vi "Form time_delays.vi"(8 "error in (no error)":errorcluster, 9 "remake":bool, 10 "Control-Client":refnum<class "Control-Client.lvclass">, 11 "Experiment in":refnum<class "Experiment.lvclass">) -> (0 "error out":errorcluster, 2 "Control-Client out":refnum<class "Control-Client.lvclass">, 3 "Experiment out":refnum<class "Experiment.lvclass">)   [LabVIEW 2018, in "Experiment.lvclass"]
uses:
  Experiment.lvclass
  Control/Control-Client/Control-Client.lvclass
  Experiment.lvclass/Experiment.ctl
  Control/Control-Client/Control-Client.lvclass/Control-Client.ctl
panel:
  out "minI":dbl
  out "Real Optical 0, ps":dbl
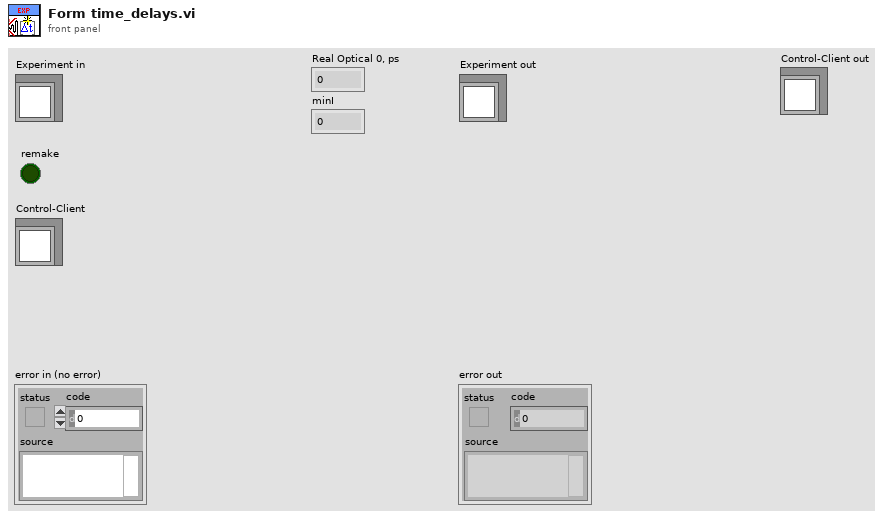
[diagram p1: front panel]
types:
  T1 = cluster{"min I, mm":dbl, "max I, mm":dbl, "Real Optical 0, ps":dbl, "min II, mm":dbl, "max II, mm ":dbl}
  T2 = typedef "Control-Client.lvclass/Delays-refs_CLIENT.ctl" = cluster{"# points":refnum<vi>, "Step, ps":refnum<vi>, "OZ, ps":refnum<vi>, "# current":refnum<vi>, "RDT, ps":refnum<vi>, "Total length, ps":refnum<vi>, "Kinetics length, ps":refnum<vi>, "Real zero, ps":refnum<vi>, "# par point":refnum<vi>}
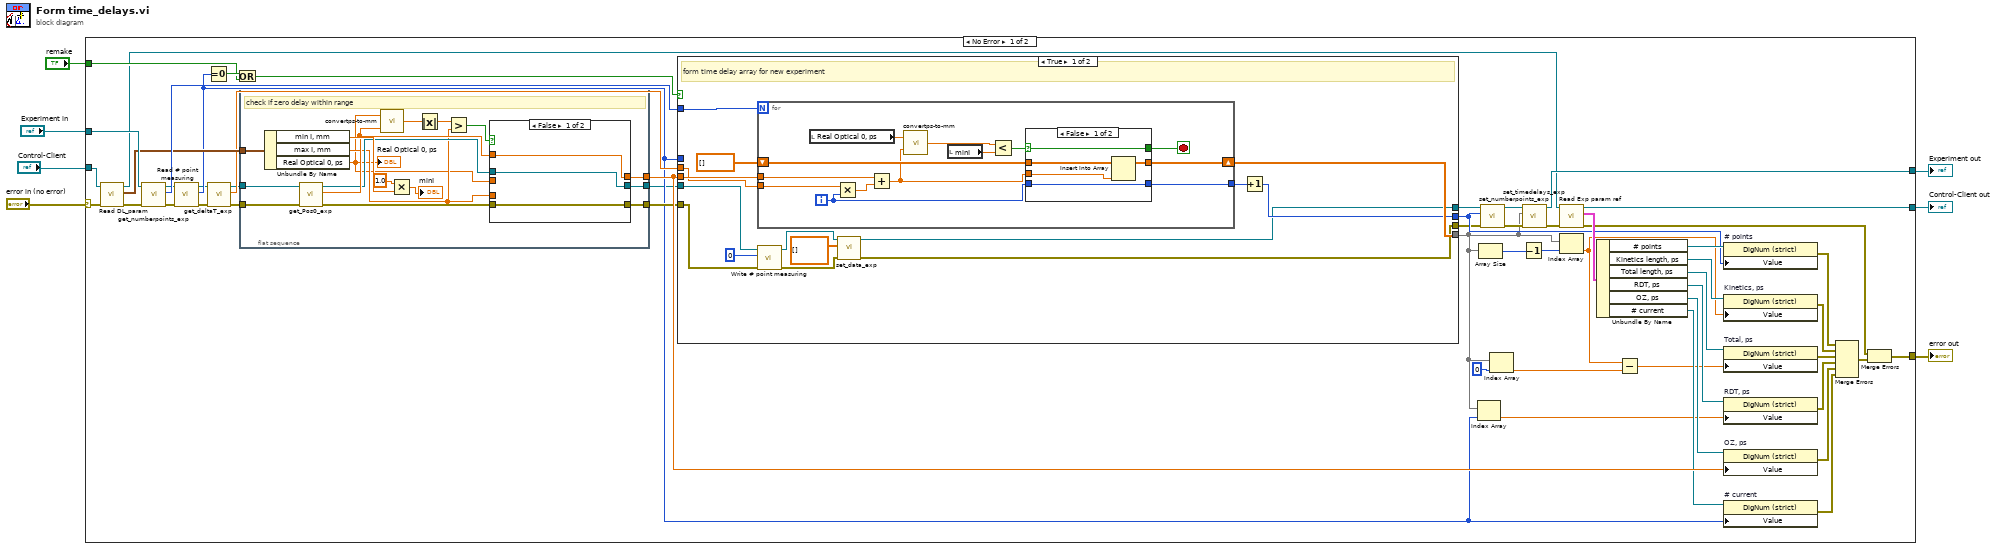
[diagram p0: block diagram]
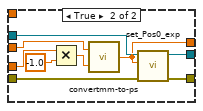
[diagram p2: hidden frame]
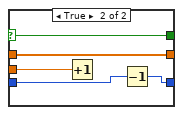
[diagram p3: hidden frame]
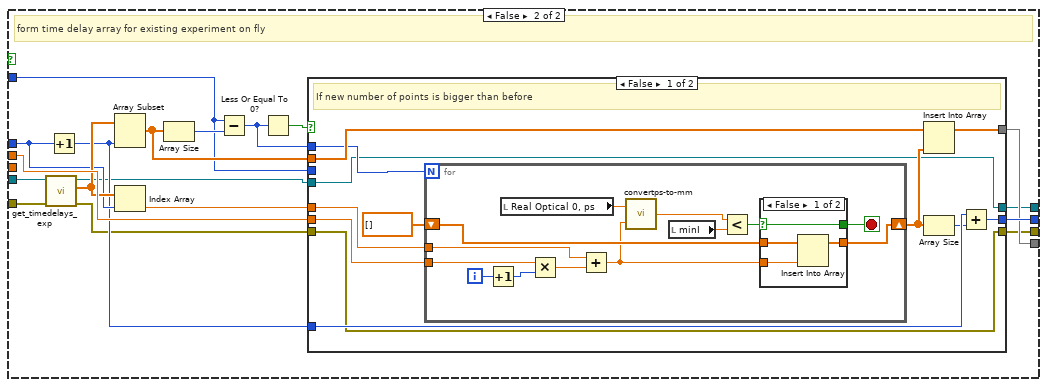
[diagram p4: hidden frame]
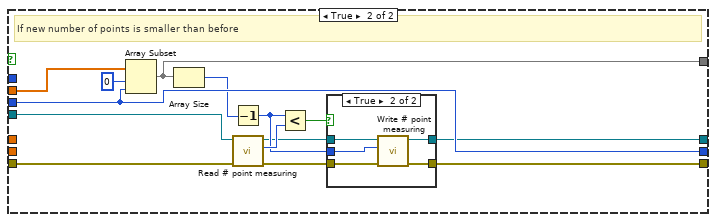
[diagram p6: hidden frame]
diagram:
  n1 = case shown="No Error" "error in (no error)" {
    selector: "error in (no error)" -> [w11 w200]
    tunnel: [w55 w200] -> w6
    tunnel: [w60 w199] -> w4
    tunnel: "Experiment in" -> [w56 w199]
    tunnel: "Control-Client" -> [w52 w198]
    tunnel: "remake" -> [w27 _]
    tunnel: [w18 w198] -> w1
    frame No Error {
      n2 = call "Read DL_param.vi"("error in (no error)"=w11, "Control-Client in"=w52) -> ("error out"=w10:errorcluster, "DL_param"=w54:T1, "Control-Client out"=w19:refnum<class "Control-Client.lvclass">)  [unwired: 7 in]
      n3 = call "get_numberpoints_exp.vi"("error in (no error)"=w10, "Experiment.lvclass in"=w56) -> ("error out"=w14:errorcluster, "numberpoints"=w59:i32, "Experiment.lvclass out"=w17:refnum<class "Experiment.lvclass">)  [unwired: 7 in]
      n4 = call "Read # point measuring.vi"("error in (no error)"=w14, "Experiment in"=w17) -> ("error out"=w13:errorcluster, "# point measuring"=w25:i32, "Experiment out"=w16:refnum<class "Experiment.lvclass">)  [unwired: 7 in]
      n5 = Equal To 0?(x=w25) -> (x = 0?=w29:bool)
      n6 = call "get_deltaT_exp.vi"("error in (no error)"=w13, "Experiment.lvclass in"=w16) -> ("error out"=w12:errorcluster, "deltaTlast"=w33:dbl, "Experiment.lvclass out"=w15:refnum<class "Experiment.lvclass">)  [unwired: 7 in]
      n7 = Or(x=w29, y=w27) -> (x .or. y?=w28:bool)
      n8 = flat-sequence {
        tunnel: w54 -> [w77]
        tunnel: [w70] -> w34
        tunnel: w15 -> [w67]
        tunnel: [w66] -> w23
        tunnel: [w63] -> w31
        tunnel: w12 -> [w61]
        frame #0 {
          # "check if zero delay within range"
          n9 = Unbundle By Name(w77) -> ("min I, mm"=w76:dbl, "max I, mm"=w65:dbl, "Real Optical 0, ps"=w64:dbl)
          "Real Optical 0, ps" <- w64
          n10 = call "get_Pos0_exp.vi"("error in (no error)"=w61, "Experiment.lvclass in"=w67) -> ("error out"=w68:errorcluster, "Delay0,ps"=w71:dbl, "Experiment.lvclass out"=w69:refnum<class "Experiment.lvclass">)  [unwired: 6 in]
          n11 = call "convertps-to-mm.vi"("ps"=w71, "Real zero"=w64) -> ("mm"=w74:dbl)
          n12 = Multiply(x=1.0, y=w76) -> (x*y=→"minI":dbl)
          n13 = Absolute Value(x=w74) -> (abs(x)=w73:dbl)
          n14 = Greater?(x=w73, y=w65) -> (0:w72:bool)
          n15 = case shown="False" w72 {
            tunnel: [w80 w83] -> w70
            tunnel: w71 -> [w80 _]
            tunnel: w69 -> [w79 w89]
            tunnel: w68 -> [w78 w88]
            tunnel: [w78 w87] -> w63
            tunnel: [w79 w86] -> w66
            tunnel: w65 -> [_ w84]
            tunnel: w64 -> [_ w85]
            frame False {
            }
            frame True {
              n16 = Multiply(x=w84, y=-1.0) -> (x*y=w82:dbl)
              n17 = call "convertmm-to-ps.vi"("mm"=w82, "Real zero"=w85) -> ("ps"=w83:dbl)
              n18 = call "set_Pos0_exp.vi"("error in (no error)"=w88, "Pos0,ps"=w83, "Experiment.lvclass in"=w89) -> ("error out"=w87:errorcluster, "Experiment.lvclass out"=w86:refnum<class "Experiment.lvclass">)  [unwired: 6 in]
            }
          }
        }
      }
      n19 = case shown="True" w28 {
        tunnel: w59 -> [w104 w134]
        tunnel: w34 -> [w103 _]
        tunnel: w33 -> [w102 w145]
        tunnel: [w98 w141] -> w50
        tunnel: [w100 w140] -> w38
        tunnel: w25 -> [_ w139]
        tunnel: w23 -> [w97 w144]
        tunnel: [w90 w131] -> w32
        tunnel: w31 -> [w96 w130]
        tunnel: [w93 w129] -> w30
        frame True {
          # "form time delay array for new experiment"
          n20 = for {
            N: w104 -> [_]
            tunnel: w103 -> [w117]
            tunnel: w102 -> [w116]
            tunnel: [w105] -> w99
            shift-right: [w107] -> w100
            shift-left: dbl[] [] ("array w/ subset deleted") -> [w109]
            i -> [w106]
            stop <- w110 stop-if-true
            n21 = local read "Real Optical 0, ps"() -> (w114:dbl)
            n22 = Multiply(x=w116, y=w106) -> (x*y=w115:dbl)
            n23 = Add(x=w117, y=w115) -> (x+y=w108:dbl)
            n24 = call "convertps-to-mm.vi"("ps"=w108, "Real zero"=w114) -> ("mm"=w113:dbl)
            n25 = local read "minI"() -> (w112:dbl)
            n26 = Less?(x=w113, y=w112) -> (x < y?=w111:bool)
            n27 = case shown="False" w111 {
              selector: w111 -> [w122 w127]
              tunnel: [w122 w127] -> w110
              tunnel: w109 -> [w121 w126]
              tunnel: w108 -> [w120 w125]
              tunnel: [w119 w126] -> w107
              tunnel: w106 -> [w118 w124]
              tunnel: [w118 w123] -> w105
              frame False {
                n28 = Insert Into Array(array=w121, new element=w120) -> (w119:dbl[])  [unwired: 1 in]
              }
              frame True {
                n29 = Increment(x=w125) -> ()  [unwired: 1 out]
                n30 = Decrement(x=w124) -> (x-1=w123:i32)
              }
            }
          }
          n31 = call "Write # point measuring.vi"("error in (no error)"=w96, "# point measuring"=0, "Experiment in"=w97) -> ("error out"=w94:errorcluster, "Experiment out"=w91:refnum<class "Experiment.lvclass">)  [unwired: 7 in]
          n32 = call "set_data_exp.vi"("error in (no error)"=w94, "Data"=dbl[][] [], "Experiment.lvclass in"=w91) -> ("error out"=w93:errorcluster, "Experiment.lvclass out"=w90:refnum<class "Experiment.lvclass">)  [unwired: 7 in]
          n33 = Increment(x=w99) -> (x+1=w98:i32)
        }
        frame False {
          # "form time delay array for existing experiment on fly"
          n34 = call "get_timedelays_exp.vi"("error in (no error)"=w130, "Experiment.lvclass in"=w144) -> ("error out"=w132:errorcluster, "timedelays"=w143:dbl[], "Experiment.lvclass out"=w133:refnum<class "Experiment.lvclass">)  [unwired: 7 in]
          n35 = Increment(x=w139) -> (x+1=w138:i32)
          n36 = Array Subset(array=w143, length=w138) -> (w137:dbl[])  [unwired: 1 in]
          n37 = Index Array(array=w143, index=w139) -> (element=w142:dbl)
          n38 = Array Size(array=w137) -> (size(s)=w136:i32)
          n39 = Subtract(x=w134, y=w136) -> (x-y=w135:i32)
          n40 = Less Or Equal To 0?(x=w135) -> (x <= 0?=w128:bool)
          n41 = case shown="False" w128 {
            tunnel: w145 -> [w157 _]
            tunnel: w142 -> [w155 _]
            tunnel: [w154 w188] -> w141
            tunnel: [w153 w186] -> w140
            tunnel: w138 -> [w152 _]
            tunnel: w137 -> [w149 w190]
            tunnel: w135 -> [w148 _]
            tunnel: w134 -> [_ w188]
            tunnel: w133 -> [w146 w187]
            tunnel: w132 -> [w147 w181]
            tunnel: [w146 w179] -> w131
            tunnel: [w147 w177] -> w129
            frame False {
              # "If new number of points is bigger than before"
              n42 = for {
                N: w148 -> [_]
                tunnel: w155 -> [w170]
                tunnel: w157 -> [w169]
                shift-right: [w160] -> w151
                shift-left: dbl[] [] -> [w162]
                i -> [w167]
                stop <- w158 stop-if-true
                n43 = Increment(x=w167) -> (x+1=w159:i32)
                n44 = local read "Real Optical 0, ps"() -> (w166:dbl)
                n45 = Multiply(x=w169, y=w159) -> (x*y=w168:dbl)
                n46 = Add(x=w170, y=w168) -> (x+y=w161:dbl)
                n47 = call "convertps-to-mm.vi"("ps"=w161, "Real zero"=w166) -> ("mm"=w165:dbl)
                n48 = local read "minI"() -> (w164:dbl)
                n49 = Less?(x=w165, y=w164) -> (x < y?=w163:bool)
                n50 = case shown="False" w163 {
                  selector: w163 -> [w174 w176]
                  tunnel: [w174 w176] -> w158
                  tunnel: w162 -> [w173 w175]
                  tunnel: w161 -> [w172 _]
                  tunnel: [w171 w175] -> w160
                  frame False {
                    n51 = Insert Into Array(array=w173, new element=w172) -> (w171:dbl[])  [unwired: 1 in]
                  }
                  frame True {
                  }
                }
              }
              n52 = Insert Into Array(array=w149, new element=w151) -> (w153:dbl[])  [unwired: 1 in]
              n53 = Array Size(array=w151) -> (size(s)=w150:i32)
              n54 = Add(x=w152, y=w150) -> (x+y=w154:i32)
            }
            frame True {
              # "If new number of points is smaller than before"
              n55 = Array Subset(array=w190, index=0, length=w188) -> (w186:dbl[])
              n56 = Array Size(array=w186) -> (size(s)=w185:i32)
              n57 = Decrement(x=w185) -> (x-1=w182:i32)
              n58 = call "Read # point measuring.vi"("error in (no error)"=w181, "Experiment in"=w187) -> ("error out"=w178:errorcluster, "# point measuring"=w184:i32, "Experiment out"=w180:refnum<class "Experiment.lvclass">)  [unwired: 7 in]
              n59 = Less?(x=w182, y=w184) -> (x < y?=w183:bool)
              n60 = case shown="True" w183 {
                tunnel: w182 -> [_ w197]
                tunnel: w180 -> [w192 w196]
                tunnel: [w192 w195] -> w179
                tunnel: w178 -> [w191 w194]
                tunnel: [w191 w193] -> w177
                frame False {
                }
                frame True {
                  n61 = call "Write # point measuring.vi"("error in (no error)"=w194, "# point measuring"=w197, "Experiment in"=w196) -> ("error out"=w193:errorcluster, "Experiment out"=w195:refnum<class "Experiment.lvclass">)  [unwired: 7 in]
                }
              }
            }
          }
        }
      }
      n62 = Index Array(array=w38, index=w25) -> (element=w22:dbl)
      n63 = Array Size(array=w38) -> (size(s)=w41:i32)
      n64 = call "set_numberpoints_exp.vi"("error in (no error)"=w30, "numberpoints"=w50, "Experiment.lvclass in"=w32) -> ("error out"=w57:errorcluster, "Experiment.lvclass out"=w58:refnum<class "Experiment.lvclass">)  [unwired: 6 in]
      n65 = Index Array(array=w38, index=0) -> (element=w37:dbl)
      n66 = Decrement(x=w41) -> (x-1=w40:i32)
      n67 = call "set_timedelays_exp.vi"("error in (no error)"=w57, "timedelays"=w38, "Experiment.lvclass in"=w58) -> ("error out"=w9:errorcluster, "Experiment.lvclass out"=w60:refnum<class "Experiment.lvclass">)  [unwired: 7 in]
      n68 = call "Read Exp param ref.vi"("error in (no error)"=w9, "Control-Client in"=w19) -> ("error out"=w8:errorcluster, "Exp param ref"=w53:T2, "Control-Client out"=w18:refnum<class "Control-Client.lvclass">)  [unwired: 7 in]
      n69 = Index Array(array=w38, index=w40) -> (element=w21:dbl)
      n70 = Unbundle By Name(w53) -> ("# points"=w51:refnum<vi>, "Kinetics length, ps"=w49:refnum<vi>, "Total length, ps"=w48:refnum<vi>, "RDT, ps"=w47:refnum<vi>, "OZ, ps"=w36:refnum<vi>, "# current"=w26:refnum<vi>)
      n71 = Subtract(x=w21, y=w37) -> (x-y=w20:dbl)
      n72 = property on="# points" class="DigNum (strict)"(reference=w51, "Value"=w50) -> (error out=w46:errorcluster)  [unwired: 1 in, 1 out]
      n73 = property on="Kinetics, ps" class="DigNum (strict)"(reference=w49, "Value"=w21) -> (error out=w45:errorcluster)  [unwired: 1 in, 1 out]
      n74 = property on="Total, ps" class="DigNum (strict)"(reference=w48, "Value"=w20) -> (error out=w44:errorcluster)  [unwired: 1 in, 1 out]
      n75 = property on="RDT, ps" class="DigNum (strict)"(reference=w47, "Value"=w22) -> (error out=w43:errorcluster)  [unwired: 1 in, 1 out]
      n76 = property on="OZ, ps" class="DigNum (strict)"(reference=w36, "Value"=w34) -> (error out=w35:errorcluster)  [unwired: 1 in, 1 out]
      n77 = property on="# current" class="DigNum (strict)"(reference=w26, "Value"=w25) -> (error out=w24:errorcluster)  [unwired: 1 in, 1 out]
      n78 = Merge Errors(w46, w45, w44, w43, w35, w24) -> (w42:errorcluster)
      n79 = Merge Errors(w8, w42) -> (w55:errorcluster)
    }
    frame Error {
    }
  }
  "error out" <- w6
  "Experiment out" <- w4
  "Control-Client out" <- w1
